vi "Begin.vi"() -> (0 "error in (no error)":errorcluster)   [LabVIEW 2014]
doc: "Called before other user functions, this VI is expected to open initial I/O refnums, load in file data, and do all program initialization. Notice that the <B>error out</B> terminal is simply used for data flow. Wiring it to other structures or subVIs ensures that this VI runs first."
uses:
  <vilib>/Rock Robotics/WPI/DriverStation/WPI_DriverStationRobotMode2.ctl
  TypeDefs/SRE Enum.ctl
  Robot Global Data.vi
  <vilib>/Rock Robotics/Network Tables/SD Write String Array.vi
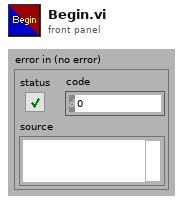
[diagram p1: front panel]
types:
  T1 = enum16{"High", "Middle", "Low", "Really Low", "Stopped"}
  T2 = enum16{"Trigger Left", "2 Left", "3 Left", "4 Left", "5 Left", "6 Left", "7 Left", "8 Left", "9 Left", "10 Left", "11 Left", "Trigger Right", "2 Right", "3 Right", "4 Right", "5 Right", "6 Right", "7 Right", "8 Right", "9 Right", "10 Right", "11 Right"}[]
  T3 = enum16{"X left ", "Y left", "Z left", "X right", "Y right", "Z right"}[]
  T4 = enum16{"A", "B", "X", "Y", "Left bumper", "Right bumper", "Back", "Start", "Left Joystick down", "Right Joystick down"}[]
  T5 = enum16{"Left X", "Left Y", "Left trigger", "R trigger", "R X", "R Y"}[]
  T6 = typedef "WPI_DriverStationRobotMode2.ctl" = enum16{"Autonomous Disabled", "Autonomous Enabled", "Teleop Disabled", "Teleop Enabled", "Disconnected", "Finish", "Test Disabled", "Test Enabled", "Emergency Stopped"}
  T7 = typedef "SRE Enum.ctl" = enum16{"Start", "Run", "End"}
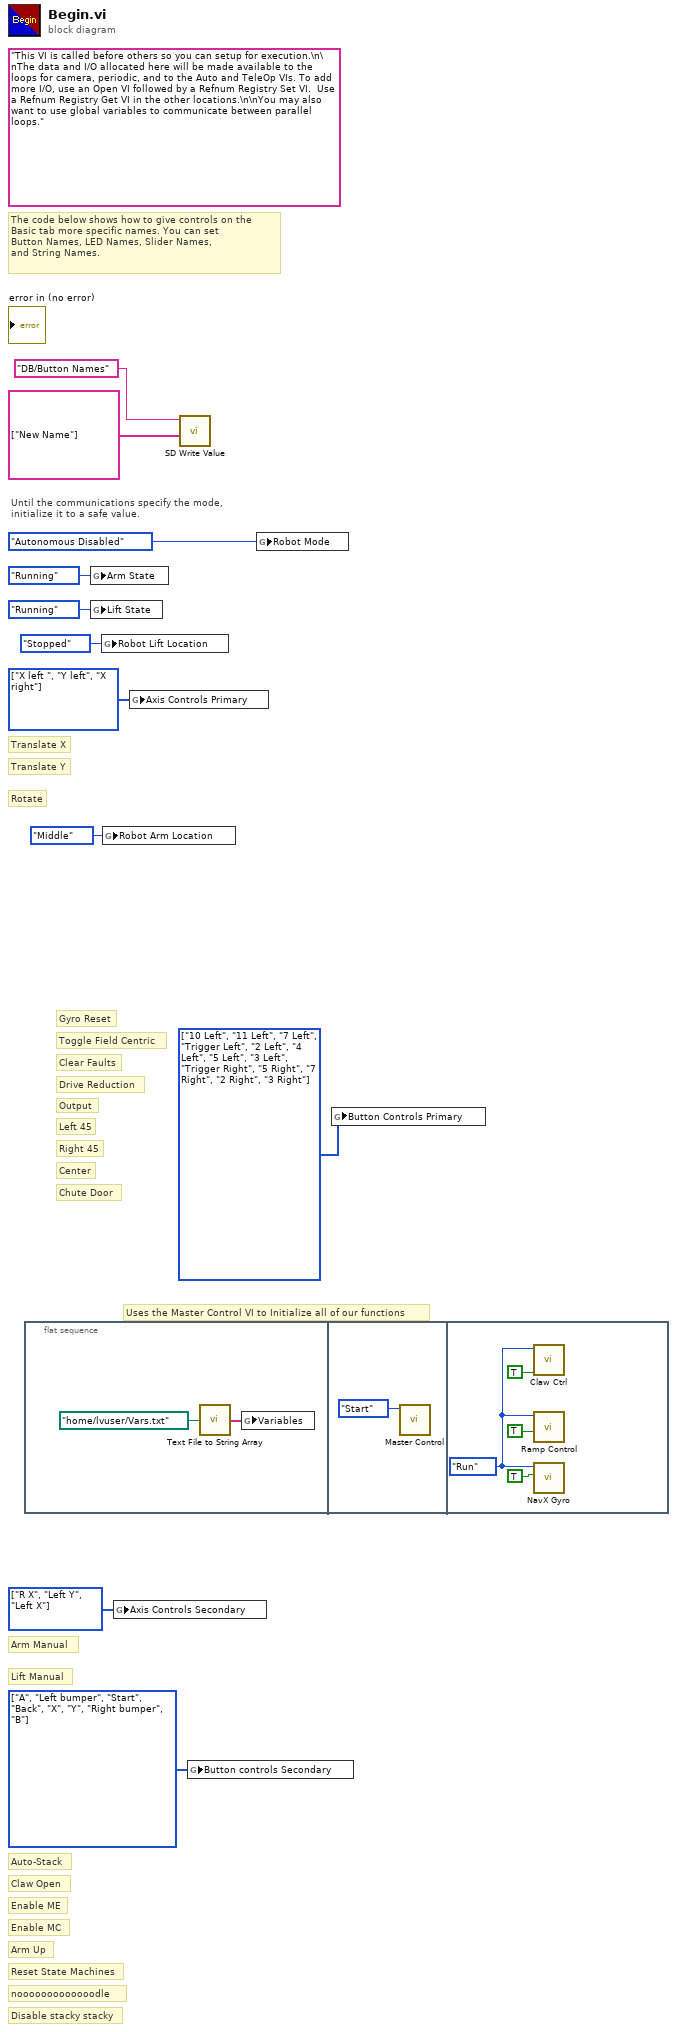
[diagram p0: block diagram]
diagram:
  w3 = T2 [enum."10 Left", enum."11 Left", enum."7 Left", enum."Trigger Left", enum."2 Left", enum."4 Left", enum."5 Left", enum."3 Left", enum."Trigger Right", enum."5 Right", enum."7 Right", enum."2 Right", enum."3 Right"] items=["Trigger Left", "2 Left", "3 Left", "4 Left", "5 Left", "6 Left", "7 Left", "8 Left", "9 Left", "10 Left", "11 Left", "Trigger Right", "2 Right", "3 Right", "4 Right", "5 Right", "6 Right", "7 Right", "8 Right", "9 Right", "10 Right", "11 Right"] ("Button Controls")
  w4 = T3 [enum."X left ", enum."Y left", enum."X right"] items=["X left ", "Y left", "Z left", "X right", "Y right", "Z right"] ("Axis Controls")
  w5 = T4 [enum."A", enum."Left bumper", enum."Start", enum."Back", enum."X", enum."Y", enum."Right bumper", enum."B"] items=["A", "B", "X", "Y", "Left bumper", "Right bumper", "Back", "Start", "Left Joystick down", "Right Joystick down"] ("Button controls Secondary")
  w8 = T5 [enum."R X", enum."Left Y", enum."Left X"] items=["Left X", "Left Y", "Left trigger", "R trigger", "R X", "R Y"] ("Axis Controls Secondary")
  (unwired) "This VI is called before others so you can setup for execution.\n\nThe data and I/O allocated here will be made available to the loops for camera, periodic, and to the Auto and TeleOp VIs. To add more I/O, use an Open VI followed by a Refnum Registry Set VI.  Use a Refnum Registry Get VI in the other locations.\n\nYou may also want to use global variables to communicate between parallel loops."
  # "Chute Door"
  # "Disable stacky stacky"
  # "nooooooooooooodle"
  # "Left 45"
  # "Right 45"
  # "Center"
  # "Reset State Machines"
  # "Arm Up"
  # "Enable MC"
  # "Enable ME"
  # "Claw Open"
  # "Output"
  # "Drive Reduction"
  # "Clear Faults"
  # "Toggle Field Centric"
  # "Gyro Reset"
  # "Rotate"
  # "Translate Y"
  # "Translate X"
  # "Auto-Stack"
  # "Lift Manual"
  # "Arm Manual"
  # "Uses the Master Control VI to Initialize all of our functions"
  # "The code below shows how to give controls on the\nBasic tab more specific names. You can set\nButton Names, LED Names, Slider Names,\nand String Names."
  # "Until the communications specify the mode,\ninitialize it to a safe value."
  n1 = flat-sequence {
    frame #0 {
      n2 = call "Text File to String Array.vi"("file (use dialog)"=path "/home/lvuser/Vars.txt") -> ("Array"=w12:string[])
      n3 = global write "Robot Global Data.vi" "Variables"(w12) -> ()
    }
    frame #1 {
      n4 = call "Master Control.vi"("Enum"=SRE_Enum."Start") -> ()  [unwired: 11 in]
    }
    frame #2 {
      w16 = SRE_Enum."Run" ("Enum")
      n5 = call "Claw Ctrl.vi"("Open/Close"=TRUE ("Reset"), "Enum"=w16) -> ()  [unwired: 10 in]
      n6 = call "Ramp Control.vi"("Forward/Reverse"=TRUE ("Reset"), "Enum"=w16) -> ()  [unwired: 9 in]
      n7 = call "NavX Gyro.vi"("Reset"=TRUE, "Enum"=w16) -> ()  [unwired: 8 in, 2 out]
    }
  }
  n8 = global write "Robot Global Data.vi" "Arm State"(enum16{"Initializing", "Running", "Manual"}."Running" ("Arm State")) -> ()
  n9 = global write "Robot Global Data.vi" "Lift State"(enum16{"Initializing", "Running", "Manual"}."Running" ("Lift State")) -> ()
  n10 = global write "Robot Global Data.vi" "Robot Lift Location"(T1."Stopped" ("Robot Lift Location")) -> ()
  n11 = global write "Robot Global Data.vi" "Robot Arm Location"(enum16{"High", "Middle", "Low", "Noodle"}."Middle" ("Robot Arm Location")) -> ()
  n12 = global write "Robot Global Data.vi" "Axis Controls Secondary"(w8) -> ()
  n13 = global write "Robot Global Data.vi" "Axis Controls Primary"(w4) -> ()
  n14 = call-poly <vilib>:"SD Write Value.vi"("String Array"=string[] ["New Name"], "Name"="DB/Button Names") -> ()  [unwired: 8 in, 2 out]
  n15 = global write "Robot Global Data.vi" "Button controls Secondary"(w5) -> ()
  n16 = global write "Robot Global Data.vi" "Robot Mode"(WPI_DriverStationRobotMode2."Autonomous Disabled" ("Robot Mode")) -> ()
  n17 = global write "Robot Global Data.vi" "Button Controls Primary"(w3) -> ()
